vi "Read Msg Input.vi"(11 "TEMPLATE Msg in":refnum<class "TEMPLATE Msg.lvclass">) -> (2 "Msg Input":refnum<class "Msg Input.lvclass">)   [LabVIEW 2025, in "_Template.lvlib" / "Templates.lvlib" / "TEMPLATE Msg.lvlib" / "TEMPLATE Msg.lvlib" / "TEMPLATE Msg.lvclass"]
uses:
  TEMPLATE Msg.lvclass
  jettl/jettl/Msg Input/Msg Input.lvclass
  TEMPLATE Msg.lvclass/TEMPLATE Msg.ctl
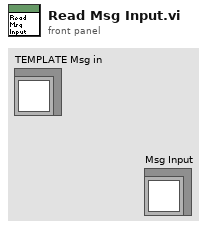
[diagram p1: front panel]
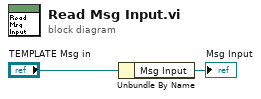
[diagram p0: block diagram]
diagram:
  n1 = Unbundle By Name("TEMPLATE Msg in") -> ("Msg Input"=→"Msg Input":refnum<class "Msg Input.lvclass">)
